vi "Read Name.vi"(8 "error in (no error)":errorcluster, 11 "Spectrometer Triax 550.lvclass in":refnum<class "Spectrometer Triax 550.lvclass">) -> (0 "error out":errorcluster, 2 "Name":string, 3 "Spectrometer Triax 550.lvclass out":refnum<class "Spectrometer Triax 550.lvclass">)   [LabVIEW 2017, in "Spectrometer Triax 550.lvclass"]
doc: "Return this Instrument's name from its member field."
uses:
  Spectrometer Triax 550.lvclass
  Utility Classes/Scannable/Scannable.lvclass
panel:
  in  "Instrument Name":string="Spectrometer Triax 550"
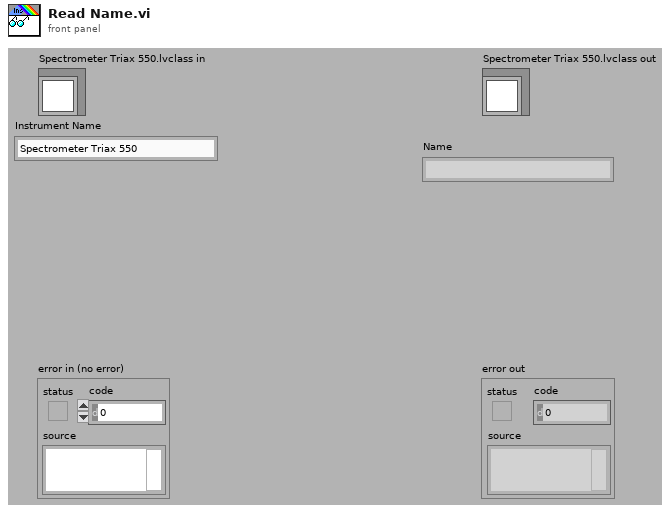
[diagram p1: front panel]
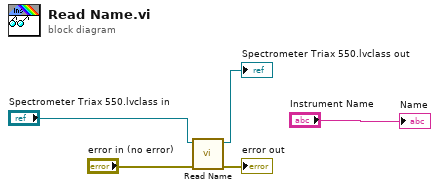
[diagram p0: block diagram]
diagram:
  n1 = call-parent "Read Name.vi"("error in (no error)"="error in (no error)", "Instrument.lvclass in"="Spectrometer Triax 550.lvclass in") -> ("error out"=→"error out":errorcluster, "Instrument.lvclass out"=→"Spectrometer Triax 550.lvclass out":refnum<class "Spectrometer Triax 550.lvclass">)  [unwired: 7 in, 1 out]
  "Name" <- "Instrument Name"
